vi "Enum to Variant Array.vi"(11 "Disabled":T1(ring)) -> (3 "Message Data Array":variant[](array[variant]))   [LabVIEW 2021, in "Game of Life.lvlib"]
doc: "Adds the Enum value as the first element of a variant array."
uses:
  Game of Life.lvlib
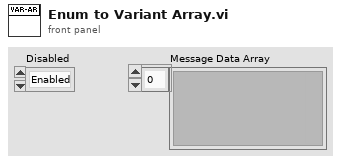
[diagram p1: front panel]
types:
  T1 = enum8{"Enabled", "Disabled", "Disabled and Grayed Out"}
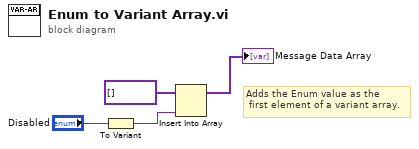
[diagram p0: block diagram]
diagram:
  # "Adds the Enum value as the\n first element of a variant array."
  n1 = To Variant(anything="Disabled") -> (Variant=w3:variant)
  n2 = Insert Into Array(array=variant[] [] ("Message Data Array"), new element=w3) -> (→"Message Data Array":variant[])  [unwired: 1 in]
